vi "FetchAllDbl.vi"(8 "error in (no error)":errorcluster, 11 "Agilent_3458 in":refnum<class "Agilent_3458.lvclass">) -> (0 "error out":errorcluster, 3 "Agilent_3458 out":refnum<class "Agilent_3458.lvclass">)   [LabVIEW 2018, in "DigitizerPlugins.lvlib" / "Agilent_3458.lvclass"]
uses:
  Agilent_3458.lvclass
  F:/Projects/ICDAS/NistPluggableModules/Digitizer/DigitizerPlugins/DigitizerBaseClass/DigitizerBase.lvclass
  DigitizerBaseClass/DigitizerBase.lvclass/DigitizerBase.ctl
  DigitizerBaseClass/Accessors/Read Handle.vi
  DigitizerBaseClass/Accessors/Read Acquisition.vi
  <instrlib>/Agilent 3458/Public/Data/Read Measurement(Multiple Points).vi
  <instrlib>/Agilent 3458/Agilent 3458.lvlib
panel:
  out "Waveform Chart":sgl[](graph)
  out "Measurements":sgl[](array[numeric])
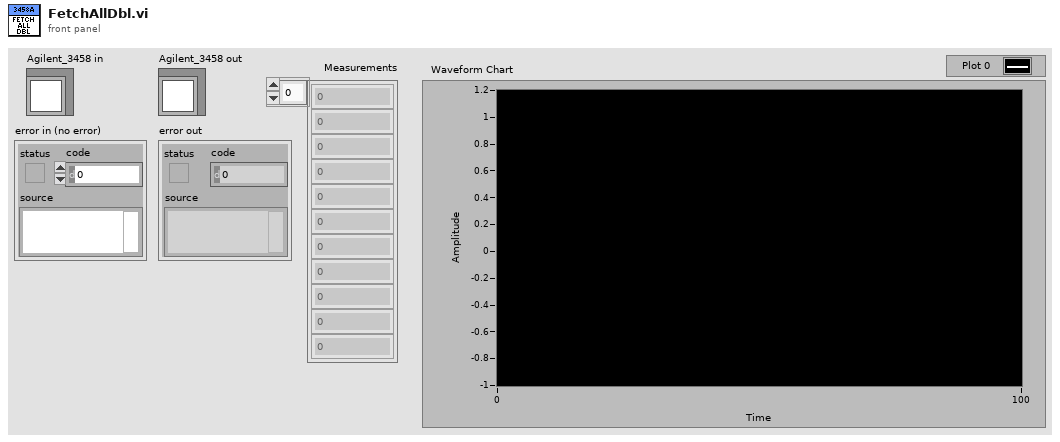
[diagram p1: front panel]
types:
  T1 = typedef "DigitizerPlugins.lvlib/DigitizerBase.lvclass/Acquisition.ctl" = cluster{"SampleRate":dbl, "RecordSize":i32, "NumRecords":i32, "SampleMode":i32, "Timeout (ms)":i32}
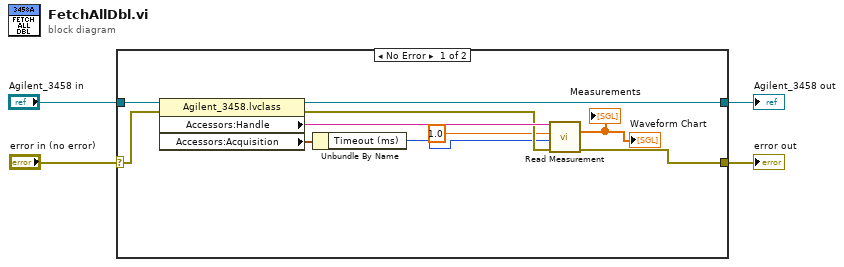
[diagram p0: block diagram]
diagram:
  n1 = case shown="No Error" "error in (no error)" {
    selector: "error in (no error)" -> [w13 w15]
    tunnel: "Agilent_3458 in" -> [w14 w16]
    tunnel: [w9 w16] -> w2
    tunnel: [w10 w15] -> w1
    frame No Error {
      n2 = property class="Agilent_3458.lvclass"(reference=w14, error in=w13) -> (reference out=w9:refnum<class "Agilent_3458.lvclass">, error out=w11:errorcluster, "Accessors:Handle"=w12:string, "Accessors:Acquisition"=w7:T1)
      n3 = Unbundle By Name(w7) -> ("Timeout (ms)"=w6:i32)
      n4 = call-poly <instrlib>:"Read Measurement.vi"("VISA resource name"=w12, "Trigger Count (1)"=1.0, "Maximum Time (10000 ms)"=w6, "error in (no error)"=w11) -> ("Measurements"=→"Measurements" →"Waveform Chart":sgl[], "error out"=w10:errorcluster)  [unwired: 9 in, 1 out]
    }
    frame Error {
    }
  }
  "error out" <- w1
  "Agilent_3458 out" <- w2
